vi "CtrlTreeAddControls.vi"(7 "Indentation":i32, 8 "error in (no error)":errorcluster, 9 "Path":string, 10 "Controls[]":refnum<vi>[](array[refnum]), 11 "TreeControl in":refnum<vi>) -> (0 "error out":errorcluster, 3 "TreeControl out":refnum<vi>)   [LabVIEW 2020]
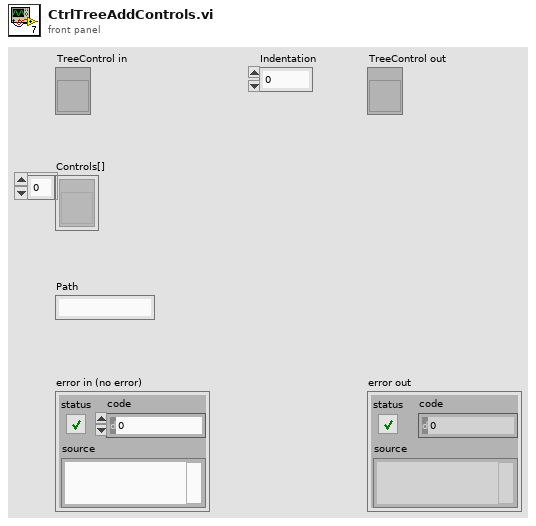
[diagram p1: front panel]
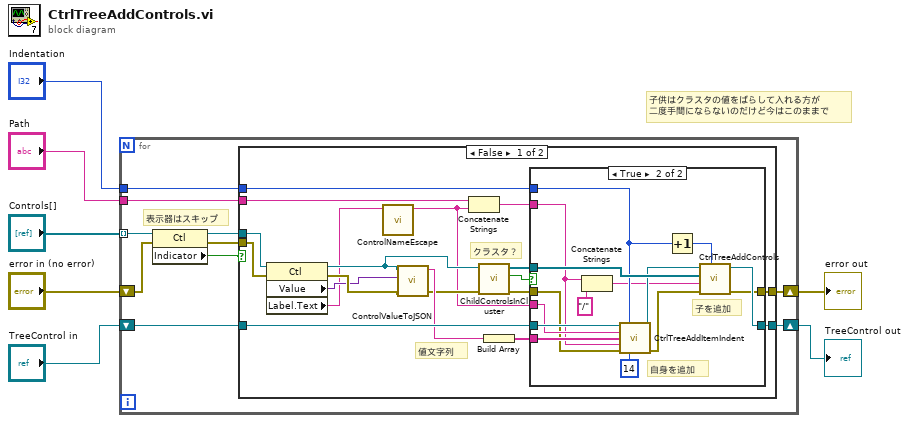
[diagram p0: block diagram]
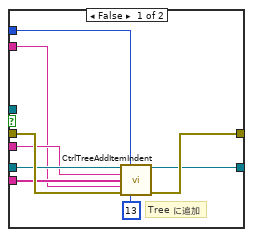
[diagram p2: hidden frame]
diagram:
  # "子供はクラスタの値をばらして入れる方が\n二度手間にならないのだけど今はこのままで"
  n1 = for {
    shift-right: [w15] -> w6
    shift-left: "TreeControl in" -> [w13]
    tunnel: "Controls[]" -> [w12] mode=indexing
    tunnel: "Path" -> [w17]
    shift-right: [w14] -> w5
    shift-left: "error in (no error)" -> [w10]
    tunnel: "Indentation" -> [w16]
    # "表示器はスキップ"
    n2 = property class="Ctl"(reference=w12, error in=w10) -> (reference out=w11:refnum<vi>, error out=w9:errorcluster, "Indicator"=w8:bool)
    n3 = case shown="False" w8 {
      tunnel: w17 -> [w36 _]
      tunnel: w16 -> [w31 _]
      tunnel: [w30 w61] -> w15
      tunnel: [w29 w62] -> w14
      tunnel: w13 -> [w28 w61]
      tunnel: w11 -> [w26 _]
      tunnel: w9 -> [w25 w62]
      frame False {
        # "値文字列"
        # "クラスタ？"
        n4 = property class="Ctl"(reference=w26, error in=w25) -> (reference out=w23:refnum<vi>, error out=w24:errorcluster, "Value"=w20:variant, "Label.Text"=w19:string)
        n5 = call "ControlNameEscape.vi"("label"=w19) -> ("escaped string"=w18:string)  [unwired: 10 in]
        n6 = call "ControlValueToJSON.vi"("error in (no error)"=w24, "Value"=w20, "Control in"=w23) -> ("error out"=w21:errorcluster, "String"=w22:string)  [unwired: 7 in]
        n7 = Concatenate Strings(w36, w18) -> (w33:string)
        n8 = call "ChildControlsInCluster.vi"("error in (no error)"=w21, "Control in"=w23) -> ("error out"=w32:errorcluster, "IsCluster"=w35:bool, "Controls[]"=w34:refnum<vi>[])  [unwired: 7 in]
        n9 = Build Array(w22) -> (w27:string[])
        n10 = case shown="True" w35 {
          tunnel: w34 -> [_ w60]
          tunnel: w33 -> [w39 w48]
          tunnel: w32 -> [w45 w51]
          tunnel: w31 -> [w38 w55]
          tunnel: [w43 w58] -> w30
          tunnel: [w44 w57] -> w29
          tunnel: w28 -> [w42 w56]
          tunnel: w18 -> [w41 w54]
          tunnel: w27 -> [w40 w53]
          frame False {
            # "Tree に追加"
            n11 = call "CtrlTreeAddItemIndent.vi"("TreeControl in"=w42, "Indentation"=w38, "Left Cell String"=w41, "Child Text"=w40, "Tag"=w39, "error in (no error)"=w45, "Symbol Index"=13) -> ("TreeControl out"=w43:refnum<vi>, "error out"=w44:errorcluster)  [unwired: 6 in, 1 out]
          }
          frame True {
            # "子を追加"
            # "自身を追加"
            n12 = Concatenate Strings(w48, "/" ("string")) -> (w47:string)
            n13 = call "CtrlTreeAddItemIndent.vi"("TreeControl in"=w56, "Indentation"=w55, "Left Cell String"=w54, "Child Text"=w53, "Tag"=w48, "error in (no error)"=w51, "Symbol Index"=14) -> ("TreeControl out"=w52:refnum<vi>, "error out"=w50:errorcluster)  [unwired: 6 in, 1 out]
            n14 = Increment(x=w55) -> (x+1=w59:i32)
            n15 = call "CtrlTreeAddControls.vi"("Indentation"=w59, "error in (no error)"=w50, "Path"=w47, "Controls[]"=w60, "TreeControl in"=w52) -> ("error out"=w57:errorcluster, "TreeControl out"=w58:refnum<vi>)  [unwired: 5 in]
          }
        }
      }
      frame True {
      }
    }
  }
  "TreeControl out" <- w6
  "error out" <- w5
